vi "vec3d to Memory Cell.vi"(10 "Vec3d in":refnum<class "Vec3d.lvclass">) -> (2 "Memory Cell":T1={"type"=enum."vector", "x"=0.0, "y"=0.0, "z"=0.0, "w"=0.0})   [LabVIEW 2024]
uses:
  Type Definitions/Memory Cell.ctl
  Type Definitions/Memory Cell Type Enum.ctl
  Shared Components/Vec3d Class/Vec3d.lvclass
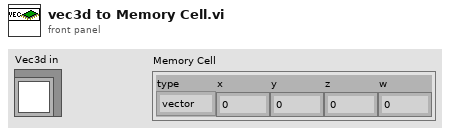
[diagram p1: front panel]
types:
  T1 = typedef "Memory Cell.ctl" = cluster{"type":T2, "x":dbl, "y":dbl, "z":dbl, "w":dbl}
  T2 = typedef "Memory Cell Type Enum.ctl" = enum16{"integer", "float", "vector", "rotation"}
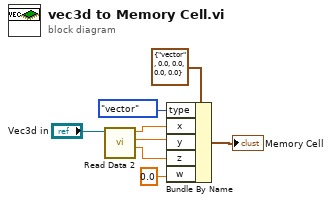
[diagram p0: block diagram]
diagram:
  n1 = call-dynamic "Read Data 2.vi"("Vec3d in"="Vec3d in") -> ("Z"=w3:dbl, "Y"=w4:dbl, "X"=w5:dbl)  [unwired: 7 in, 1 out]
  n2 = Bundle By Name(cluster=T1 {"type"=enum."vector", "x"=0.0, "y"=0.0, "z"=0.0, "w"=0.0} ("Memory Cell 2"), "type"=Memory_Cell_Type_Enum."vector", "x"=w5, "y"=w4, "z"=w3, "w"=0.0) -> (→"Memory Cell":T1)
